vi "SLM_control_v5.vi"() -> ()   [LabVIEW 2023]
panel:
  out "error out":errorcluster
  in  "Modulation Depth":dbl=214.0
  in  "SLM Monitor":i32=2
  in  "Correction Pattern":path
  in  "SLM Size":i32=800
  in  "Initialize SLM":bool
  in  "Continuous Button":bool
  in  "Single Upload":bool
  out "SLM Final Phase":dbl[][](graph)
  in  "MegaPixels Y":i32=4
  in  "MegaPixels X":i32=4
  in  "Grating Sliders":cluster{"Y":sgl, "X":sgl} {"X" min=0 max=10 step=0.01 scale=0.0..10.0; "Y" min=0 max=10 step=0.01 scale=0.0..10.0}
  in  "Phase Array":dbl[][](array[numeric])
  in  "Start/Stop":bool
  out "Phase Array Graph":dbl[][](graph)
  # "X"
  # "Y"
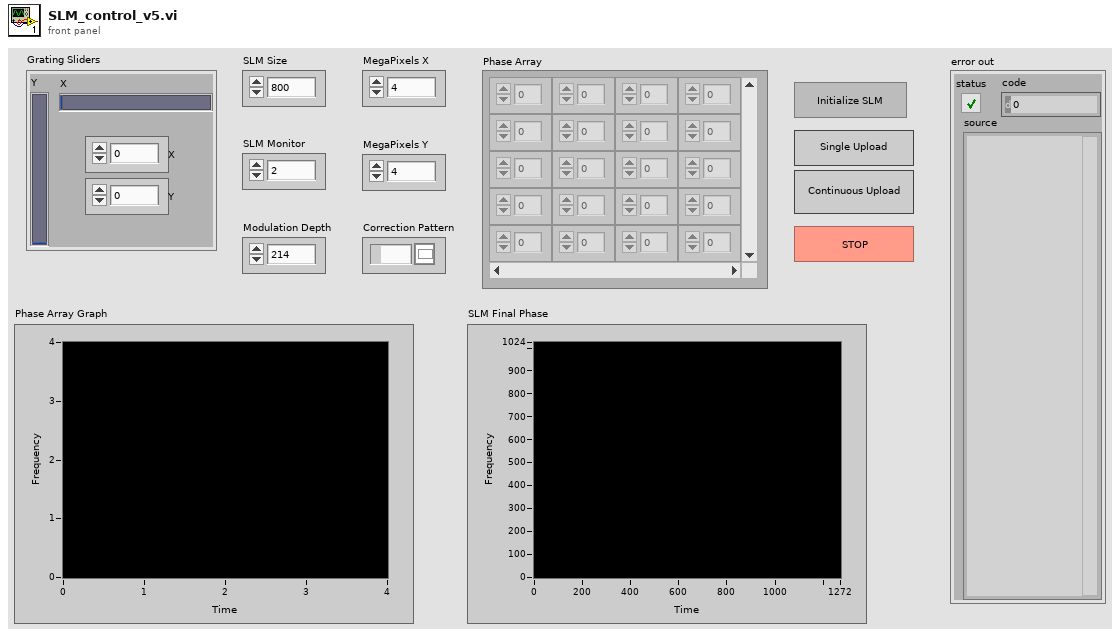
[diagram p1: front panel]
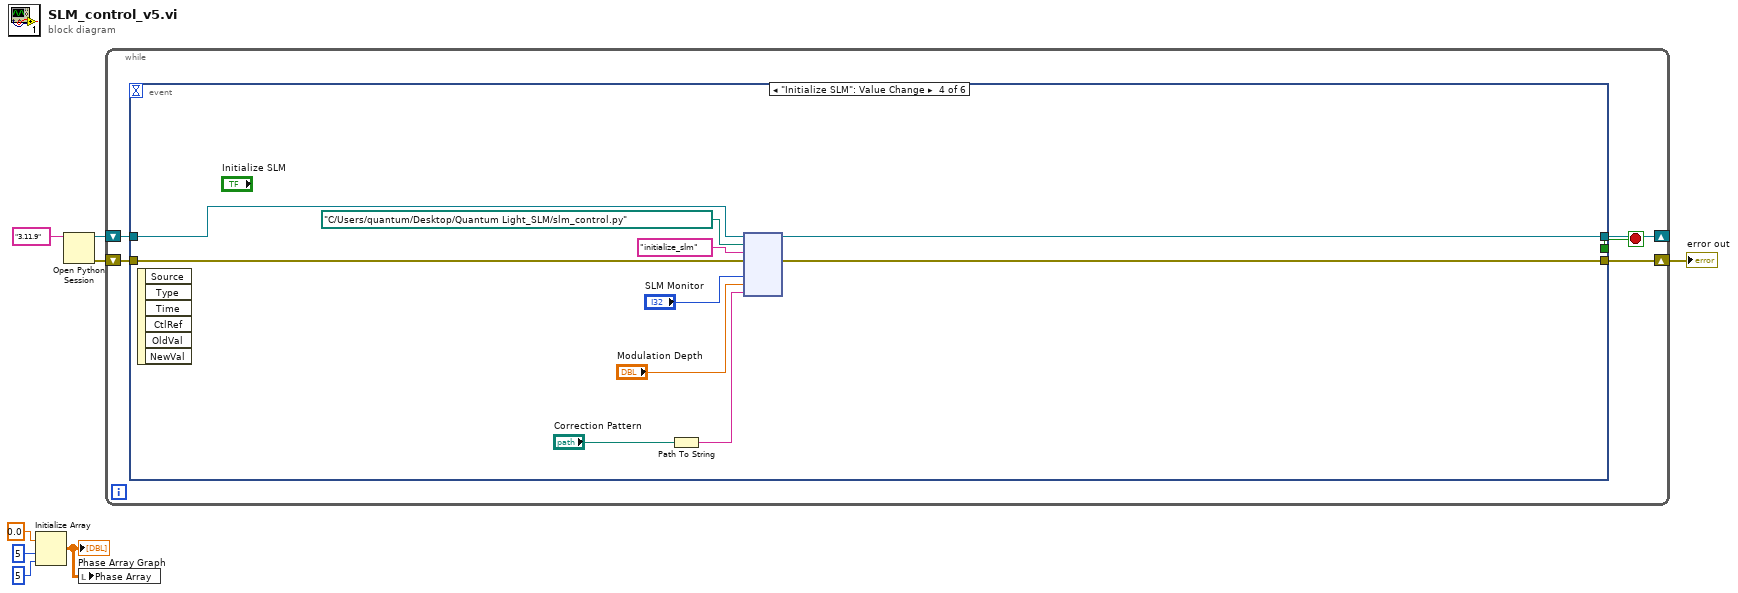
[diagram p0: block diagram]
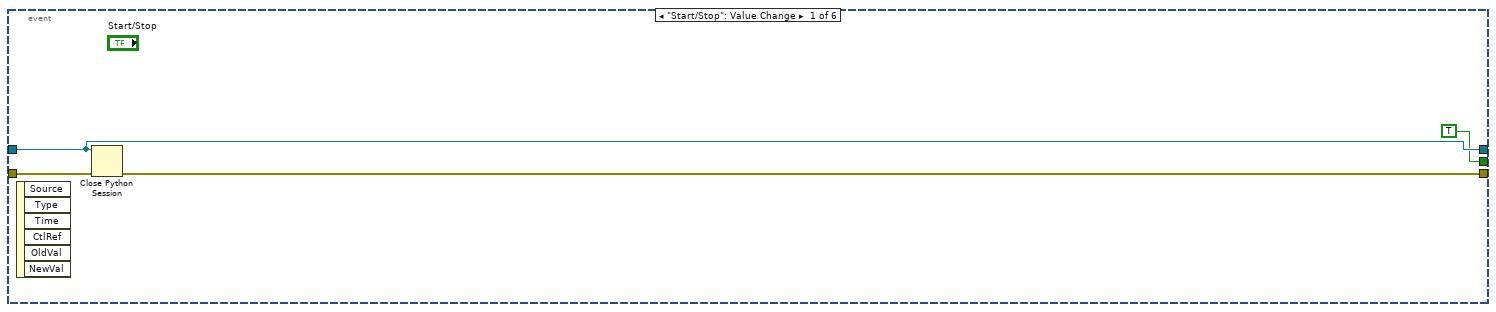
[diagram p2: hidden frame]
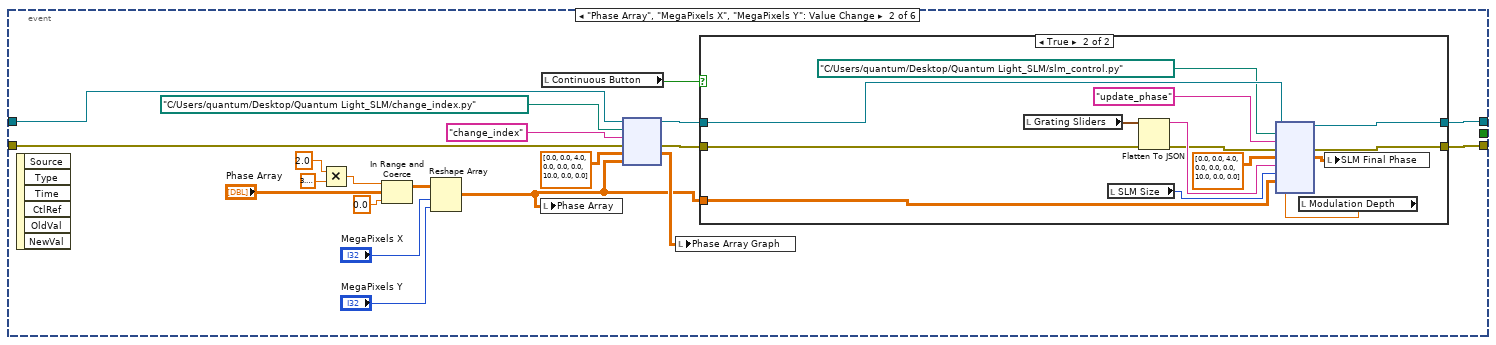
[diagram p3: hidden frame]
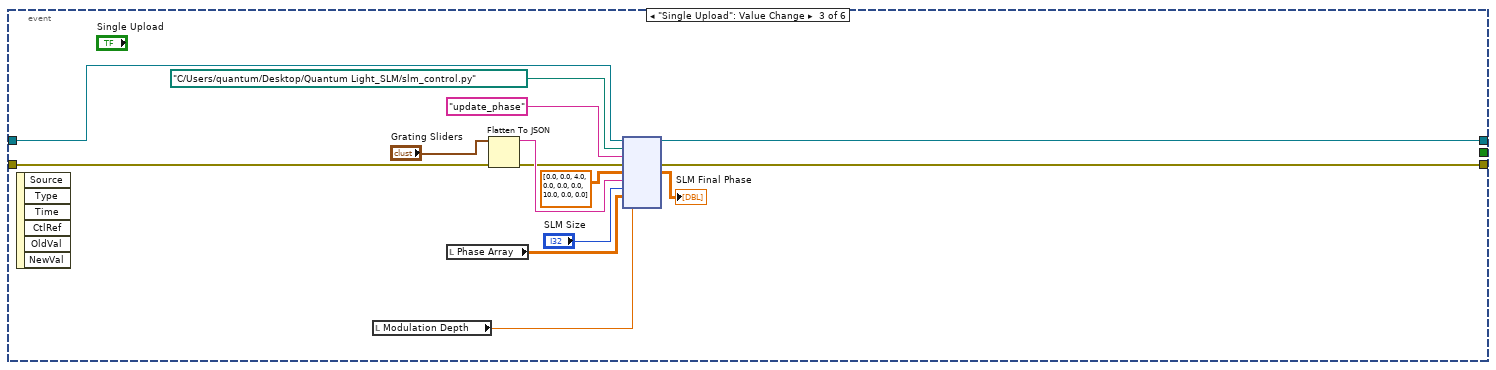
[diagram p5: hidden frame]
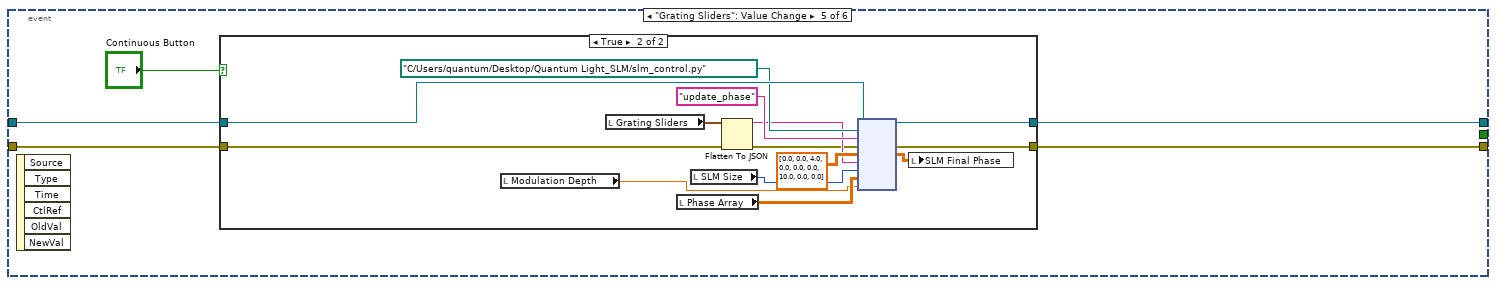
[diagram p6: hidden frame]
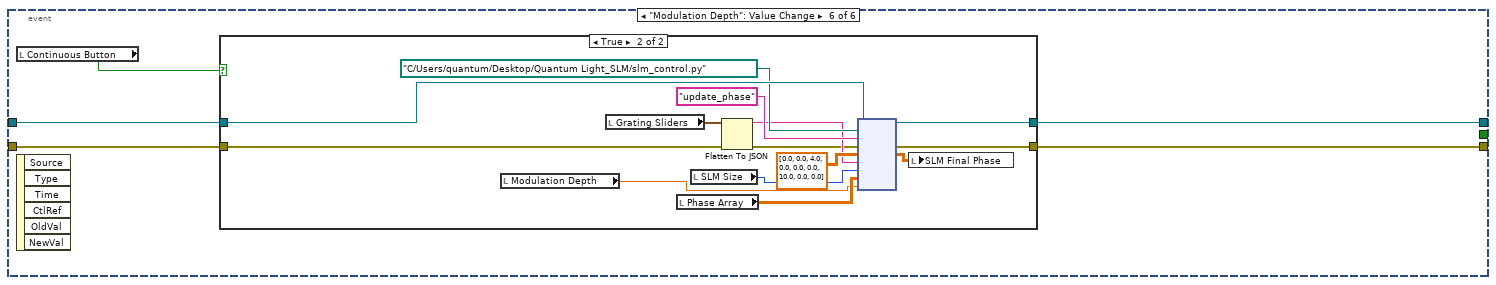
[diagram p8: hidden frame]
diagram:
  n1 = Initialize Array(0.0 ("element"), 5 ("dimension size"), 5 ("dimension size")) -> (w2:dbl[][])
  "Phase Array Graph" <- w2
  n2 = Open Python Session(python version="3.11.9" ("Python version")) -> (session out=w8:refnum<k35>, error out=w7:errorcluster)  [unwired: 2 in]
  n3 = local write "Phase Array"(w2) -> ()
  n4 = while {
    shift-right: [w10] -> _
    shift-left: w8 -> [w13]
    shift-right: [w11] -> w1
    shift-left: w7 -> [w12]
    stop <- w9 stop-if-true
    n5 = event shown="[3] \"Initialize SLM\": Value Change" {
      selector: _ -> [_ _ _ _ _ _]
      dyn-events: _ -> [_ _ _ _ _ _]
      timeout: _ -> [_ _ _ _ _ _]
      tunnel: w13 -> [w15 w31 w67 w77 w82 w103]
      tunnel: w12 -> [w17 w30 w56 w76 w81 w102]
      tunnel: [w16 w20 w65 w74 w79 w100] -> w11
      tunnel: [w15 w21 w66 w75 w80 w101] -> w10
      tunnel: [TRUE ("Start/Stop") _ _ _ _ _] -> w9
      event "Start/Stop": Value Change {
        n6 = event-data() -> ()  [unwired: 1 in, 6 out]
        n7 = Close Python Session(session in=w15, error in=w17) -> (11:w16:errorcluster)
      }
      event "Phase Array", "MegaPixels X", "MegaPixels Y": Value Change {
        n8 = event-data() -> ()  [unwired: 1 in, 6 out]
        n9 = Multiply(x=2.0, y=3.141592653589793) -> (x*y=w35:dbl)
        n10 = In Range and Coerce(upper limit=w35, x="Phase Array", lower limit=0.0) -> (coerced(x)=w36:dbl[][])  [unwired: 1 out]
        n11 = Reshape Array "Reshape Array"(w36, "MegaPixels X", "MegaPixels Y") -> (w18:dbl[][])
        n12 = local write "Phase Array"(w18) -> ()
        n13 = local read "Continuous Button"() -> (w22:bool)
        n14 = node(w31, path "C:/Users/quantum/Desktop/Quantum Light_SLM/change_index.py" ("module path"), "change_index" ("function name"), w30, dbl[][] [[0.0, 0.0, 4.0], [0.0, 0.0, 0.0], [10.0, 0.0, 0.0]] ("Python Graph"), w18) -> (w23:refnum<k35>, w24:errorcluster, w19:dbl[][])  [unwired: 1 in, 2 out]
        n15 = local write "Phase Array Graph"(w19) -> ()
        n16 = case shown="True" w22 {
          tunnel: w23 -> [w38 w53]
          tunnel: w24 -> [w39 w43]
          tunnel: [w38 w52] -> w21
          tunnel: [w39 w51] -> w20
          tunnel: w18 -> [_ w41]
          frame False {
          }
          frame True {
            n17 = local read "Grating Sliders"() -> (w45:cluster{"Y":sgl, "X":sgl})
            n18 = local read "SLM Size"() -> (w46:i32)
            n19 = Flatten To JSON(anything=w45, error in (no error)=w43) -> (JSON string=w44:string, 11:w42:errorcluster)  [unwired: 1 in]
            n20 = local read "Modulation Depth"() -> (w40:dbl)
            n21 = node(w53, path "C:/Users/quantum/Desktop/Quantum Light_SLM/slm_control.py" ("module path"), "update_phase" ("function name"), w42, dbl[][] [[0.0, 0.0, 4.0], [0.0, 0.0, 0.0], [10.0, 0.0, 0.0]] ("Python Graph"), w44, w46, w41, w40) -> (w52:refnum<k35>, w51:errorcluster, w47:dbl[][])  [unwired: 4 in, 2 out]
            n22 = local write "SLM Final Phase"(w47) -> ()
          }
        }
      }
      event "Single Upload": Value Change {
        n23 = event-data() -> ()  [unwired: 1 in, 6 out]
        n24 = local read "Modulation Depth"() -> (w54:dbl)
        n25 = local read "Phase Array"() -> (w60:dbl[][])
        n26 = Flatten To JSON(anything="Grating Sliders", error in (no error)=w56) -> (JSON string=w57:string, 11:w55:errorcluster)  [unwired: 1 in]
        n27 = node(w67, path "C:/Users/quantum/Desktop/Quantum Light_SLM/slm_control.py" ("module path"), "update_phase" ("function name"), w55, dbl[][] [[0.0, 0.0, 4.0], [0.0, 0.0, 0.0], [10.0, 0.0, 0.0]] ("Python Graph"), w57, "SLM Size", w60, w54) -> (w66:refnum<k35>, w65:errorcluster, →"SLM Final Phase":dbl[][])  [unwired: 4 in, 2 out]
      }
      event "Initialize SLM": Value Change {
        n28 = event-data() -> ()  [unwired: 1 in, 6 out]
        n29 = Path To String(path="Correction Pattern") -> (string=w69:string)
        n30 = node(w77, path "C:/Users/quantum/Desktop/Quantum Light_SLM/slm_control.py" ("module path"), "initialize_slm" ("function name"), w76, "SLM Monitor", "Modulation Depth", w69) -> (w75:refnum<k35>, w74:errorcluster)  [unwired: 5 in, 2 out]
      }
      event "Grating Sliders": Value Change {
        n31 = event-data() -> ()  [unwired: 1 in, 6 out]
        n32 = case shown="True" "Continuous Button" {
          tunnel: w82 -> [w83 w98]
          tunnel: w81 -> [w84 w87]
          tunnel: [w83 w97] -> w80
          tunnel: [w84 w96] -> w79
          frame False {
          }
          frame True {
            n33 = local read "Modulation Depth"() -> (w85:dbl)
            n34 = local read "Grating Sliders"() -> (w89:cluster{"Y":sgl, "X":sgl})
            n35 = local read "Phase Array"() -> (w91:dbl[][])
            n36 = local read "SLM Size"() -> (w90:i32)
            n37 = Flatten To JSON(anything=w89, error in (no error)=w87) -> (JSON string=w88:string, 11:w86:errorcluster)  [unwired: 1 in]
            n38 = node(w98, path "C:/Users/quantum/Desktop/Quantum Light_SLM/slm_control.py" ("module path"), "update_phase" ("function name"), w86, dbl[][] [[0.0, 0.0, 4.0], [0.0, 0.0, 0.0], [10.0, 0.0, 0.0]] ("Python Graph"), w88, w90, w91, w85) -> (w97:refnum<k35>, w96:errorcluster, w92:dbl[][])  [unwired: 4 in, 2 out]
            n39 = local write "SLM Final Phase"(w92) -> ()
          }
        }
      }
      event "Modulation Depth": Value Change {
        n40 = local read "Continuous Button"() -> (w99:bool)
        n41 = event-data() -> ()  [unwired: 1 in, 6 out]
        n42 = case shown="True" w99 {
          tunnel: w103 -> [w104 w119]
          tunnel: w102 -> [w105 w108]
          tunnel: [w104 w118] -> w101
          tunnel: [w105 w117] -> w100
          frame False {
          }
          frame True {
            n43 = local read "Modulation Depth"() -> (w106:dbl)
            n44 = local read "Grating Sliders"() -> (w110:cluster{"Y":sgl, "X":sgl})
            n45 = local read "Phase Array"() -> (w112:dbl[][])
            n46 = local read "SLM Size"() -> (w111:i32)
            n47 = Flatten To JSON(anything=w110, error in (no error)=w108) -> (JSON string=w109:string, 11:w107:errorcluster)  [unwired: 1 in]
            n48 = node(w119, path "C:/Users/quantum/Desktop/Quantum Light_SLM/slm_control.py" ("module path"), "update_phase" ("function name"), w107, dbl[][] [[0.0, 0.0, 4.0], [0.0, 0.0, 0.0], [10.0, 0.0, 0.0]] ("Python Graph"), w109, w111, w112, w106) -> (w118:refnum<k35>, w117:errorcluster, w113:dbl[][])  [unwired: 4 in, 2 out]
            n49 = local write "SLM Final Phase"(w113) -> ()
          }
        }
      }
    }
  }
  "error out" <- w1
